vi "Ke2000 Reading.vi"(8 "error in (no error)":errorcluster, 11 "VISA resource name":refnum<visa-resource-name>) -> (0 "error out":errorcluster, 1 "Units":string, 2 "Measurement":dbl, 3 "VISA resource name out":refnum<visa-resource-name>)   [LabVIEW 2012]
panel:
  out "Channel":i32
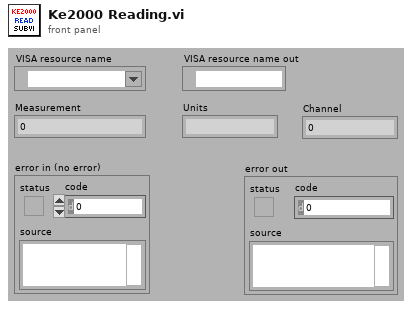
[diagram p1: front panel]
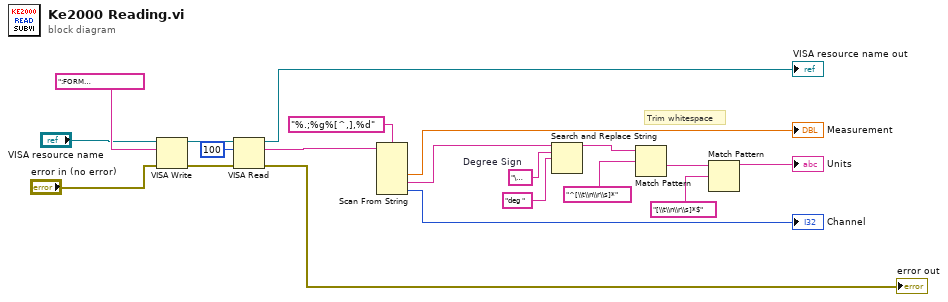
[diagram p0: block diagram]
diagram:
  w5 = "\u0013"  # Degree Sign
  # "Trim whitespace"
  n1 = VISA Write(VISA resource name="VISA resource name", write buffer=":FORM ASC;:FORM:ELEM READ,UNIT,CHAN;:SENS:DATA?", error in (no error)="error in (no error)") -> (VISA resource name out=w19:refnum<visa-resource-name>, error out=w18:errorcluster)  [unwired: 1 out]
  n2 = VISA Read(VISA resource name=w19, byte count=u32 100, error in (no error)=w18) -> (VISA resource name out=→"VISA resource name out":refnum<visa-resource-name>, read buffer=w3:string, error out=→"error out":errorcluster)  [unwired: 1 out]
  n3 = Scan From String(format string="%.;%g%[^,],%d", input string=w3) -> (output 1=→"Measurement":dbl, output 2=w6:string, output 3=→"Channel":i32)  [unwired: 5 in, 3 out]
  n4 = Search and Replace String(input string=w6, search string=w5, replace string="deg " ("replace string (\"\")")) -> (result string=w13:string)  [unwired: 5 in, 3 out]
  n5 = Match Pattern(string=w13, regular expression="^[\\t\\n\\r\\s]*") -> (after substring=w10:string)  [unwired: 1 in, 3 out]
  n6 = Match Pattern(string=w10, regular expression="[\\t\\n\\r\\s]*$") -> (before substring=→"Units":string)  [unwired: 1 in, 3 out]
